vi "save_tiff.vi"(8 "error in (no error)":errorcluster, 10 "Data":dbl[][](array[numeric]), 11 "Path":string) -> (0 "error out":errorcluster)   [LabVIEW 2011, in "Fiberscope_library.lvlib"]
uses:
  Fiberscope_library.lvlib
  common/libraries/TIFFManagement/VisualCPP/Release/TIFFManagement.dll
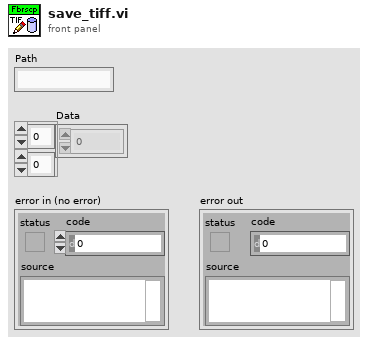
[diagram p1: front panel]
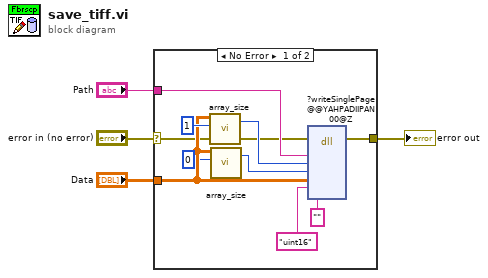
[diagram p0: block diagram]
diagram:
  n1 = case shown="No Error" "error in (no error)" {
    selector: "error in (no error)" -> [w5 w15]
    tunnel: [w14 w15] -> w4
    tunnel: "Path" -> [w13 _]
    tunnel: "Data" -> [w10 _]
    frame No Error {
      n2 = call "array_size.vi"("Array"=w10, "Dimension"=1) -> ("Dimension size"=w12:i32)  [unwired: 4 in]
      n3 = call "array_size.vi"("Array"=w10, "Dimension"=0) -> ("Dimension size"=w9:i32)  [unwired: 4 in]
      n4 = dll-call lib="C:/helioscan/common/libraries/TIFFManagement/VisualCPP/Release/TIFFManagement.dll" fn="?writeSinglePage@@YAHPADIIPAN00@Z"(error in=w5, "path"=w13, "width"=w12, "height"=w9, "data"=w10, "format"="uint16", "description"="") -> (error out=w14:errorcluster)  [unwired: 9 in, 1 out]
    }
    frame Error {
    }
  }
  "error out" <- w4
